vi "Read from Hardware.vi"(8 "error in":errorcluster, 10 "values in":dbl[](array[numeric]), 11 "triggers execution unit":refnum<class "Triggers Execution Unit.lvclass">) -> (0 "error out":errorcluster, 2 "values out":dbl[](array[numeric]), 3 "triggers execution unit out":refnum<class "Triggers Execution Unit.lvclass">)   [LabVIEW 2020, in "AIM MIL-STD-1553 Engine.lvlib" / "Implementation.lvlib" / "Triggers Execution Unit.lvclass"]
uses:
  Triggers Execution Unit.lvclass
  Triggers Execution Unit.lvclass/Triggers Execution Unit.ctl
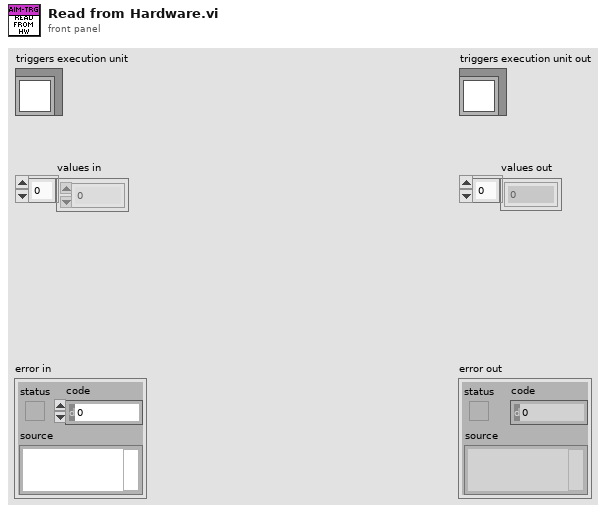
[diagram p1: front panel]
types:
  T1 = typedef "Running Status.ctl" = enum16{"Running", "Stopped"}
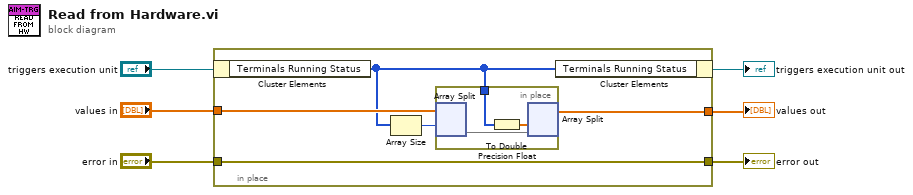
[diagram p0: block diagram]
diagram:
  n1 = in-place {
    in-place-border: "values in" -> [w10]
    in-place-border: "error in" -> [w11]
    in-place-border: [w11] -> w2
    in-place-border: [w7] -> w1
    n2 = in-place-cluster #1("triggers execution unit") -> ("Terminals Running Status"=w8:T1[])
    n3 = Array Size(array=w8) -> (size(s)=w9:i32)
    n4 = in-place {
      in-place-border: w8 -> [w14]
      n5 = in-place-split #2(w10, w9) -> (w12:dbl[])  [unwired: 1 out]
      n6 = To Double Precision Float(number=w14) -> (double precision float=w13:dbl[])
      n7 = in-place-split #2(w13, w12) -> (w7:dbl[])  [unwired: 1 out]
    }
    n8 = in-place-cluster #1("Terminals Running Status"=w8) -> (→"triggers execution unit out":refnum<class "Triggers Execution Unit.lvclass">)
  }
  "error out" <- w2
  "values out" <- w1
